vi "SIM Clock Period From Stepsize.vi"(10 "Clock Rate (Hz)":u32, 11 "Step Size":dbl) -> (2 "Valid?":bool, 3 "Period":i64=1 min=1)   [LabVIEW 2017]
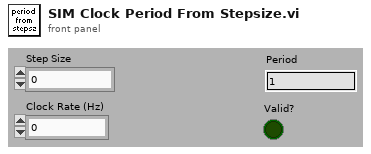
[diagram p1: front panel]
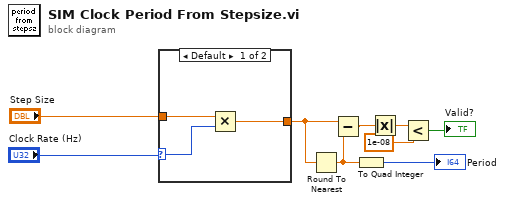
[diagram p0: block diagram]
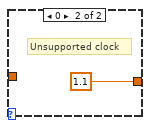
[diagram p2: hidden frame]
diagram:
  n1 = case shown="Default" "Clock Rate (Hz)" {
    selector: "Clock Rate (Hz)" -> [w10 _]
    tunnel: "Step Size" -> [w12 _]
    tunnel: [w11 1.1] -> w3
    frame Default {
      n2 = Multiply(x=w12, y=w10) -> (x*y=w11:dbl)
    }
    frame 0 {
      # "Unsupported clock"
    }
  }
  n3 = Round To Nearest(number=w3) -> (nearest integer value=w2:dbl)
  n4 = Subtract(x=w3, y=w2) -> (x-y=w7:dbl)
  n5 = To Quad Integer(1:w2) -> (0:→"Period":i64)
  n6 = Absolute Value(x=w7) -> (abs(x)=w6:dbl)
  n7 = Less?(x=w6, y=1e-08) -> (x < y?=→"Valid?":bool)
